vi "stristr.vi"(3 "offset (0)":i32, 4 "Substring":string="CDE", 5 "Input String":string="abcdef") -> (0 "offset of match":i32=-99, 1 "found":bool, 2 "match + rest of string":string)   [LabVIEW 2020]
doc: "Finds the first occurrence of a substring in a string (ignoring case). The \"offset of match\" is the position of search the string/char in the input string. The offset of the first character in a string is zero. The \"offset of match\" is -1 if no match is found."
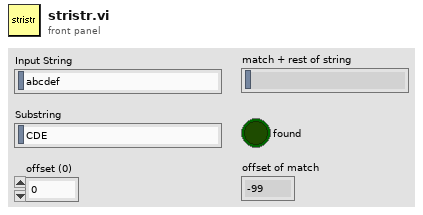
[diagram p1: front panel]
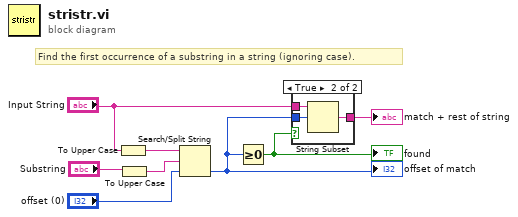
[diagram p0: block diagram]
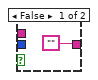
[diagram p2: hidden frame]
diagram:
  # "Find the first occurrence of a substring in a string (ignoring case)."
  n1 = To Upper Case(1:"Input String") -> (0:w8:string)
  n2 = To Upper Case(1:"Substring") -> (0:w6:string)
  n3 = Search/Split String(string=w8, search string/char (-)=w6, offset (0)="offset (0)") -> (offset of match=w2:i32)  [unwired: 2 out]
  "offset of match" <- w2
  n4 = Greater Or Equal To 0?(x=w2) -> (x >= 0?=w1:bool)
  "found" <- w1
  n5 = case shown="True" w1 {
    tunnel: ["" w12] -> w5
    tunnel: "Input String" -> [_ w11]
    tunnel: w2 -> [_ w10]
    frame False {
    }
    frame True {
      n6 = String Subset(string=w11, offset (0)=w10) -> (substring=w12:string)  [unwired: 1 in]
    }
  }
  "match + rest of string" <- w5
